vi "cost_subvi.vi"() -> (0 "capirinha":dbl format="%.2f", 1 "Whisky-sour":dbl format="%.2f", 2 "Whisky-cola":dbl format="%.2f", 3 "Whater-juice":dbl format="%.2f", 4 "Water":dbl format="%.2f", 5 "Cola":dbl format="%.2f")   [LabVIEW 2019]
uses:
  <vilib>/Utility/config.llb/Read Key (Double).vi
  <vilib>/Utility/config.llb/NI_LVConfig.lvlib
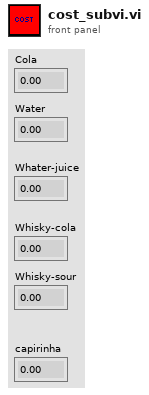
[diagram p1: front panel]
types:
  T1 = typedef "NI_LVConfig.lvlib/Config Data RefNum.ctl" = refnum<k1>
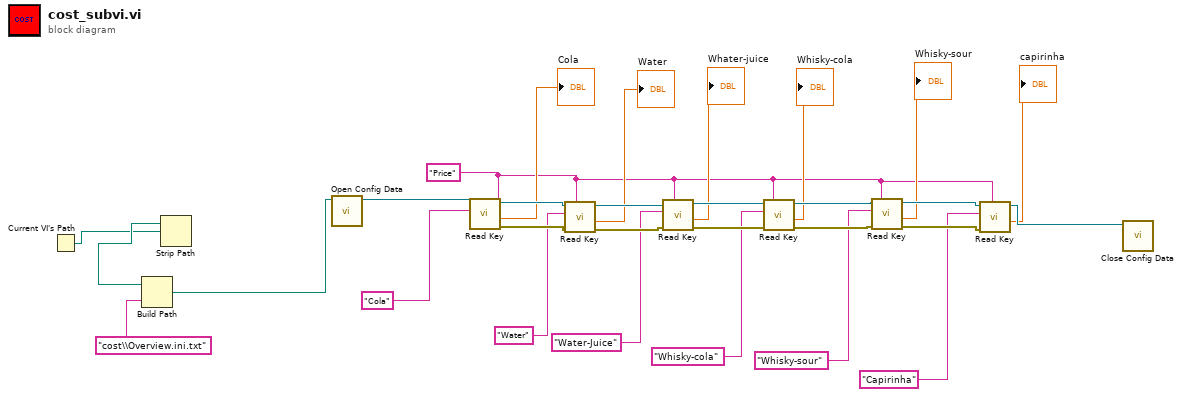
[diagram p0: block diagram]
diagram:
  w11 = "Price" ("section")
  n1 = Current VI's Path() -> (path=w2:path)
  n2 = Strip Path(path=w2) -> (stripped path=w4:path)  [unwired: 1 out]
  n3 = Build Path(base path=w4, name or relative path="cost\\Overview.ini.txt") -> (appended path=w1:path)
  n4 = call <vilib>:"Open Config Data.vi"("configuration file path"=w1) -> ("refnum"=w29:T1)  [unwired: 8 in, 2 out]
  n5 = call-poly <vilib>:"Read Key.vi"("section"=w11, "key"="Cola", "refnum"=w29) -> ("error out"=w22:errorcluster, "value"=→"Cola":dbl, "refnum out"=w28:T1)  [unwired: 5 in, 1 out]
  n6 = call-poly <vilib>:"Read Key.vi"("section"=w11, "error in (no error)"=w22, "key"="Water", "refnum"=w28) -> ("error out"=w21:errorcluster, "value"=→"Water":dbl, "refnum out"=w27:T1)  [unwired: 4 in, 1 out]
  n7 = call-poly <vilib>:"Read Key.vi"("section"=w11, "error in (no error)"=w21, "key"="Water-Juice", "refnum"=w27) -> ("error out"=w20:errorcluster, "value"=→"Whater-juice":dbl, "refnum out"=w26:T1)  [unwired: 4 in, 1 out]
  n8 = call-poly <vilib>:"Read Key.vi"("section"=w11, "error in (no error)"=w20, "key"="Whisky-cola", "refnum"=w26) -> ("error out"=w19:errorcluster, "value"=→"Whisky-cola":dbl, "refnum out"=w25:T1)  [unwired: 4 in, 1 out]
  n9 = call-poly <vilib>:"Read Key.vi"("section"=w11, "error in (no error)"=w19, "key"="Whisky-sour", "refnum"=w25) -> ("error out"=w18:errorcluster, "value"=→"Whisky-sour":dbl, "refnum out"=w24:T1)  [unwired: 4 in, 1 out]
  n10 = call-poly <vilib>:"Read Key.vi"("section"=w11, "error in (no error)"=w18, "key"="Capirinha", "refnum"=w24) -> ("value"=→"capirinha":dbl, "refnum out"=w23:T1)  [unwired: 4 in, 2 out]
  n11 = call <vilib>:"Close Config Data.vi"("refnum"=w23) -> ()  [unwired: 9 in, 2 out]
